vi "Read Actual Transition Time.vi"(8 "error in (no error)":errorcluster, 11 "signal configuration in":refnum<class "SV Signal.lvclass">) -> (0 "error out":errorcluster, 2 "actual transition time":dbl, 3 "signal configuration out":refnum<class "SV Signal.lvclass">)   [LabVIEW 2017, in "SV Signal.lvclass"]
uses:
  <vilib>/addons/_NISVFA/_Generation/Signal Generation/SV Signal/SV Signal.lvclass
  <vilib>/addons/_NISVFA/_Generation/Signal Generation/SV Signal/sv_Signal State Attribute.ctl
  <vilib>/addons/_NISVFA/_Generation/Signal Generation/SV Signal/SV Signal.lvclass/SV Signal.ctl
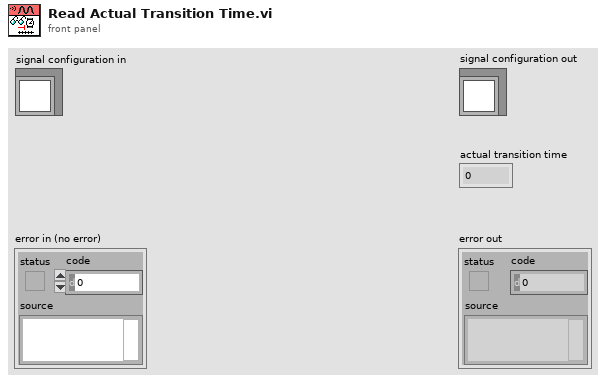
[diagram p1: front panel]
types:
  T1 = typedef "SV Signal.lvclass/sv_Signal State Attribute.ctl" = string
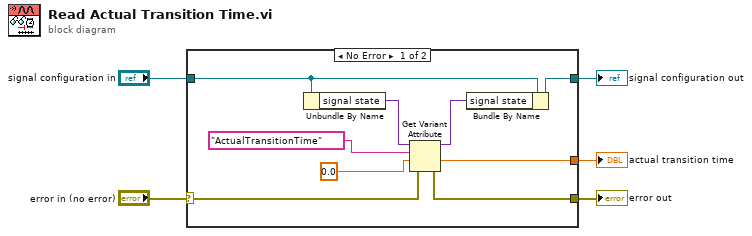
[diagram p0: block diagram]
diagram:
  n1 = case shown="No Error" "error in (no error)" {
    selector: "error in (no error)" -> [w10 w16]
    tunnel: [w9 w16] -> w4
    tunnel: [w11 w15] -> w2
    tunnel: "signal configuration in" -> [w12 w15]
    tunnel: [w6 _] -> w1
    frame No Error {
      n2 = Unbundle By Name(w12) -> ("signal state"=w13:variant)
      n3 = Get Variant Attribute(Variant=w13, name=T1 "ActualTransitionTime" ("attribute"), default value (empty Variant)=0.0 ("actual transition time"), error in=w10) -> (duplicate Variant=w14:variant, value=w6:dbl, error out=w9:errorcluster)  [unwired: 1 out]
      n4 = Bundle By Name(cluster=w12, "signal state"=w14) -> (w11:refnum<class "SV Signal.lvclass">)
    }
    frame Error {
    }
  }
  "error out" <- w4
  "signal configuration out" <- w2
  "actual transition time" <- w1
